vi "02grabareeprom.vi"(1 "Pagina 2":string, 2 "Pagina 1":string, 3 "timeout ms (500)":i32=500, 4 "Puerto":u16, 5 "address":string) -> (0 "Error?":bool)   [LabVIEW 2010]
panel:
  out "error out":errorcluster
  out "ID in":refnum<k5>
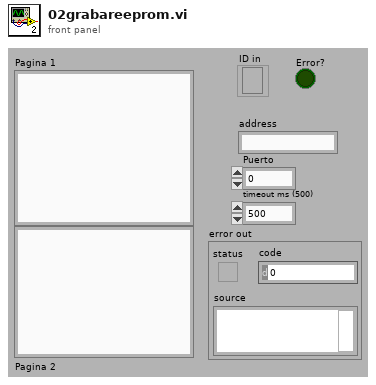
[diagram p1: front panel]
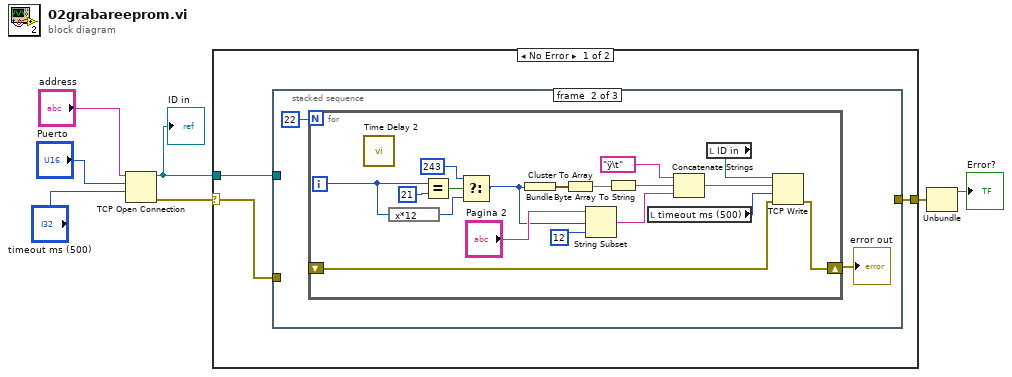
[diagram p0: block diagram]
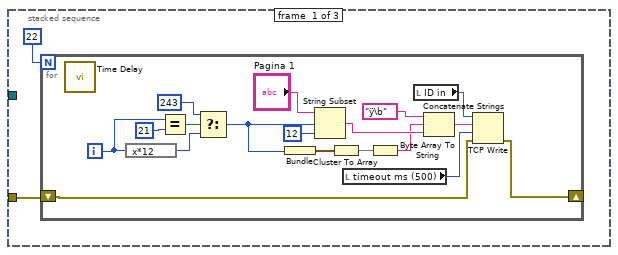
[diagram p2: hidden frame]
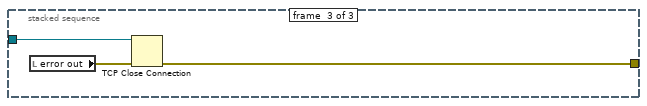
[diagram p3: hidden frame]
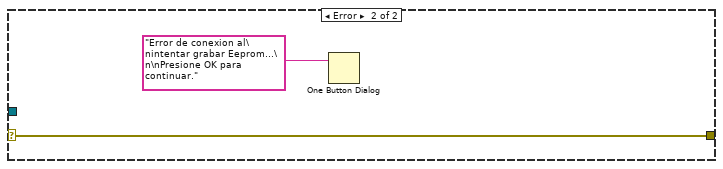
[diagram p4: hidden frame]
diagram:
  n1 = TCP Open Connection(address="address", remote port or service name="Puerto", timeout ms (60000)="timeout ms (500)") -> (connection ID=w3:refnum<k5>, error out=w6:errorcluster)  [unwired: 1 in, 1 out]
  "ID in" <- w3
  n2 = case shown="No Error" w6 {
    selector: w6 -> [w8 w54]
    tunnel: w3 -> [w10 _]
    tunnel: [w9 w54] -> w2
    frame No Error {
      n3 = stacked-sequence {
        tunnel: w10 -> [_ _ w53]
        tunnel: [_ _ w52] -> w9
        tunnel: w8 -> [w11 _ _]
        frame #0 {
          n4 = for {
            N: 22 ("Numeric") -> [_]
            shift-right: [w20] -> _
            shift-left: w11 -> [w19]
            i -> [w16]
            n5 = call "Time Delay"() -> ()  [unwired: 2 in, 10 out]
            n6 = expression code="x*12"(w16) -> (w14:i32)
            n7 = Equal?(x=w16, y=21) -> (x = y?=w18:bool)
            n8 = Select(t=243, s=w18, f=w14) -> (s? t:f=w13:i32)
            n9 = Bundle(w13) -> (w27:cluster{i32})  [unwired: 1 in]
            n10 = String Subset(string="Pagina 1", offset (0)=w13, length (rest)=12 ("length (rest)")) -> (substring=w30:string)
            n11 = Cluster To Array(cluster=w27) -> (array=w26:i32[])
            n12 = local read "timeout ms (500)"() -> (w21:i32)
            n13 = Byte Array To String(unsigned byte array=w26) -> (string=w25:string)
            n14 = local read "ID in"() -> (w23:refnum<k5>)
            n15 = Concatenate Strings("ÿ\b" ("string"), w25, w30) -> (w24:string)
            n16 = TCP Write(connection ID=w23, data in=w24, error in (no error)=w19, 9:w21) -> (error out=w20:errorcluster)  [unwired: 2 out]
          }
        }
        frame #1 {
          n17 = for {
            N: 22 -> [_]
            shift-right: [w40] -> w31
            shift-left: _ -> [w39]
            i -> [w33]
            n18 = call "Time Delay 2"() -> ()  [unwired: 2 in, 10 out]
            n19 = expression code="x*12"(w33) -> (w35:i32)
            n20 = Equal?(x=w33, y=21) -> (x = y?=w38:bool)
            n21 = Select(t=243, s=w38, f=w35) -> (s? t:f=w34:i32)
            n22 = Bundle(w34) -> (w47:cluster{i32})  [unwired: 1 in]
            n23 = Cluster To Array(cluster=w47) -> (array=w46:i32[])
            n24 = String Subset(string="Pagina 2", offset (0)=w34, length (rest)=12 ("length (rest)")) -> (substring=w50:string)
            n25 = Byte Array To String(unsigned byte array=w46) -> (string=w45:string)
            n26 = local read "timeout ms (500)"() -> (w41:i32)
            n27 = Concatenate Strings("ÿ\t" ("string"), w45, w50) -> (w44:string)
            n28 = local read "ID in"() -> (w43:refnum<k5>)
            n29 = TCP Write(connection ID=w43, data in=w44, error in (no error)=w39, 9:w41) -> (error out=w40:errorcluster)  [unwired: 2 out]
          }
          "error out" <- w31
        }
        frame #2 {
          n30 = local read "error out"() -> (w51:errorcluster)
          n31 = TCP Close Connection(connection ID=w53, error in (no error)=w51) -> (error out=w52:errorcluster)  [unwired: 2 out]
        }
      }
    }
    frame Error {
      n32 = One Button Dialog(message="Error de conexion al\nintentar grabar Eeprom...\n\nPresione OK para continuar.") -> ()  [unwired: 2 out]
    }
  }
  n33 = Unbundle(w2) -> ("status"=→"Error?":bool)  [unwired: 2 out]
